vi "Start_Client.vi"   [LabVIEW 2020]
uses:
  Database/Global1.vi
types:
  T1 = cluster{"设备名称":string, "操作人员":string, "设备状态":enum16{"设备离线", "设备正常", "设备缺料", "设备故障", "质量报警"}, "附加信息":string}
  T2 = enum32{"Invalid", "Standard", "Closed", "Hidden", "Minimized", "Maximized"}
  T3 = cluster{"用户编号":string, "用户名":string, "用户密码(密文)":string, "用户权限":string}
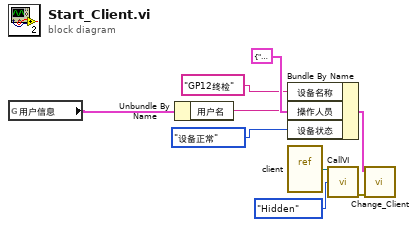
[diagram p0: block diagram]
diagram:
  n1 = global read "Global1.vi" "用户信息"() -> (w1:T3)
  n2 = Unbundle By Name(w1) -> ("用户名"=w3:string)
  n3 = Bundle By Name(cluster=T1 {"设备名称"="", "操作人员"="", "设备状态"=enum."设备离线", "附加信息"=""} ("设备信息"), "设备名称"="GP12终检", "操作人员"=w3, "设备状态"=enum16{"设备离线", "设备正常", "设备缺料", "设备故障", "质量报警"}."设备正常") -> (w2:T1)
  n4 = vi-ref "client.vi"() -> (w9:refnum<vi>)
  n5 = call "CallVI.vi"("VI引用"=w9, "状态"=T2."Hidden") -> ("错误输出"=w7:errorcluster)  [unwired: 11 in, 2 out]
  n6 = call "Change_Client.vi"("错误输入（无错误）"=w7, "设备信息"=w2) -> ()  [unwired: 9 in, 1 out]
